vi "Problemas_Monitoreo_03.vi"() -> ()   [LabVIEW 2020]
uses:
  <vilib>/Instr/_visa.llb/VISA Configure Serial Port (Instr).vi
panel:
  in  "stop":bool
  in  "VISA resource name":refnum<visa-resource-name>
  out "concatenated string":string
  in  "string":string
  out "concatenated string 2":string
  in  "Boolean":bool
  in  "Boolean 2":bool
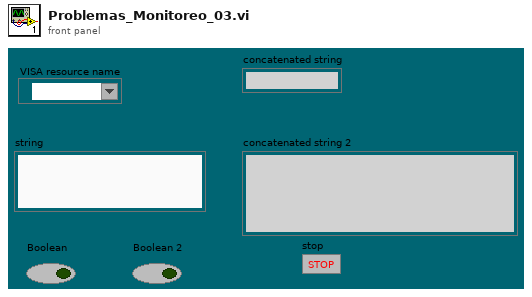
[diagram p1: front panel]
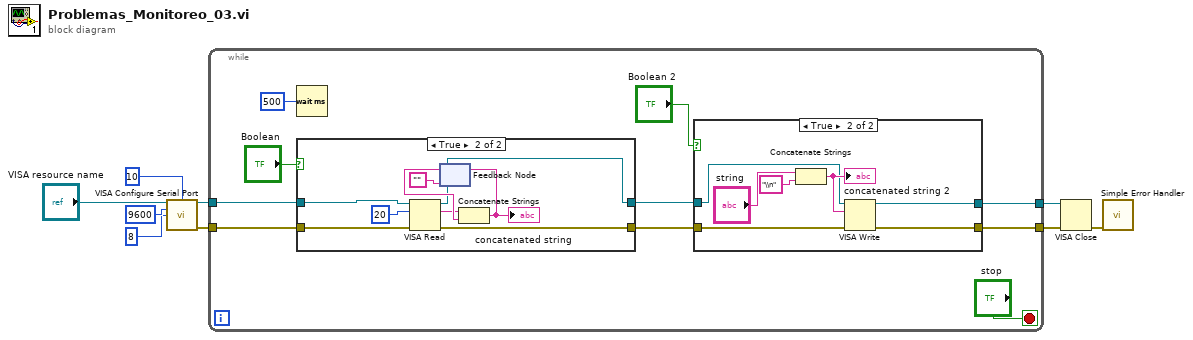
[diagram p0: block diagram]
diagram:
  n1 = call-poly "VISA Configure Serial Port"("VISA resource name"="VISA resource name", "termination char\n(0xA = '\\n' = LF)"=u8 10 ("termination char\n(0xA = '\\n' = LF)"), "baud rate (9600)"=u32 9600, "data bits (8)"=u16 8) -> ("VISA resource name out"=w4:refnum<visa-resource-name>, "error out"=w3:errorcluster)  [unwired: 10 in]
  n2 = while {
    tunnel: w4 -> [w17]
    tunnel: w3 -> [w15]
    tunnel: [w11] -> w2
    tunnel: [w12] -> w1
    stop <- "stop" stop-if-true
    n3 = Wait (ms)(milliseconds to wait=u32 500) -> ()  [unwired: 1 out]
    n4 = case shown="True" "Boolean" {
      tunnel: w17 -> [w30 w34]
      tunnel: [w29 w33] -> w14
      tunnel: [w30 w32] -> w13
      tunnel: w15 -> [w29 w31]
      frame False {
      }
      frame True {
        n5 = VISA Read(VISA resource name=w34, byte count=u32 20, error in (no error)=w31) -> (VISA resource name out=w32:refnum<visa-resource-name>, read buffer=w37:string, error out=w33:errorcluster)  [unwired: 1 out]
        n6 = feedback #1("") -> (w39:string)
        n7 = Concatenate Strings(w37, w39) -> (w38:string)
        "concatenated string" <- w38
        n8 = feedback-in #1(w38) -> ()
      }
    }
    n9 = case shown="True" "Boolean 2" {
      tunnel: w14 -> [w21 w25]
      tunnel: w13 -> [w20 w24]
      tunnel: [w21 w23] -> w12
      tunnel: [w20 w22] -> w11
      frame False {
      }
      frame True {
        n10 = Concatenate Strings("string", "\\n" ("string")) -> (w27:string)
        "concatenated string 2" <- w27
        n11 = VISA Write(VISA resource name=w24, write buffer=w27, error in (no error)=w25) -> (VISA resource name out=w22:refnum<visa-resource-name>, error out=w23:errorcluster)  [unwired: 1 out]
      }
    }
  }
  n12 = VISA Close(VISA resource name=w2, error in (no error)=w1) -> (error out=w6:errorcluster)
  n13 = call <vilib>:"Simple Error Handler.vi"("error in (no error)"=w6) -> ()  [unwired: 4 in, 5 out]
